vi "Intan_Update_XY_AxisLims.vi"(0 "NscansRead":i32, 1 "offset factor":dbl=1.0, 5 "FS (Hz)":dbl, 7 "XscaleClusterCurrent":T1, 9 "DisplayLength(s)":dbl, 11 "DT_scale (s)":dbl, 12 "Nchans to Display":i16) -> (4 "XscaleRollover":bool, 6 "DispLengthChanged":bool, 8 "offsetChanged":bool, 10 "NchansChanged":bool, 14 "XYlims Update Cluster":T2, 15 "UpdateCode":i16)   [LabVIEW 2017]
panel:
  out "Nupdates":dbl
  out "samps displayed":i64
  out "newXoffset":dbl
  out "YscaleMinOut":dbl
  out "YscaleMax_Out":dbl
  out "XscaleOffsetOut":dbl
  out "XscaleMaxOut":dbl
  out "XscaleMinOut":dbl
  out "Time since last update (s)":dbl
  out "NsampsSinceScrnUpdate":i64
  out "Nsamps refresh":dbl
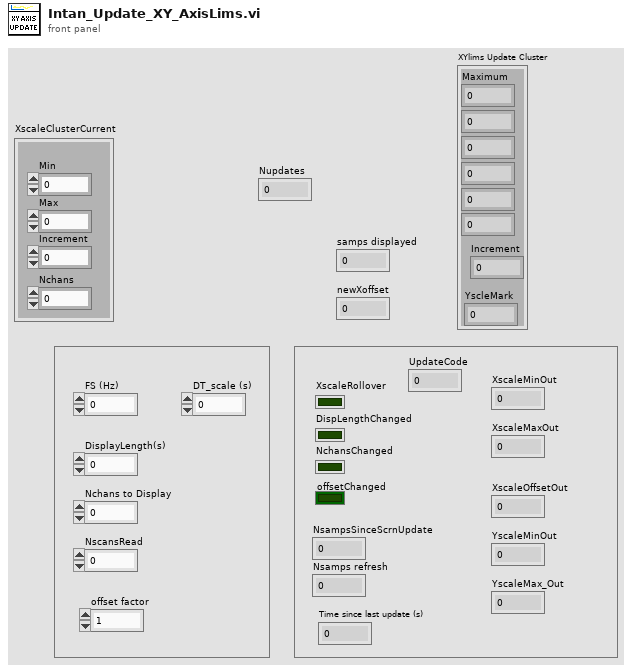
[diagram p1: front panel]
types:
  T1 = cluster{"Min":dbl, "Max":dbl, "Increment":dbl, "Nchans":dbl}
  T2 = cluster{"Maximum":dbl, dbl, dbl, dbl, dbl, dbl, "YscleMark":dbl, "Increment":dbl}
  T3 = cluster{"Max":dbl, dbl, dbl, dbl, dbl, dbl, dbl, "Increment":dbl}
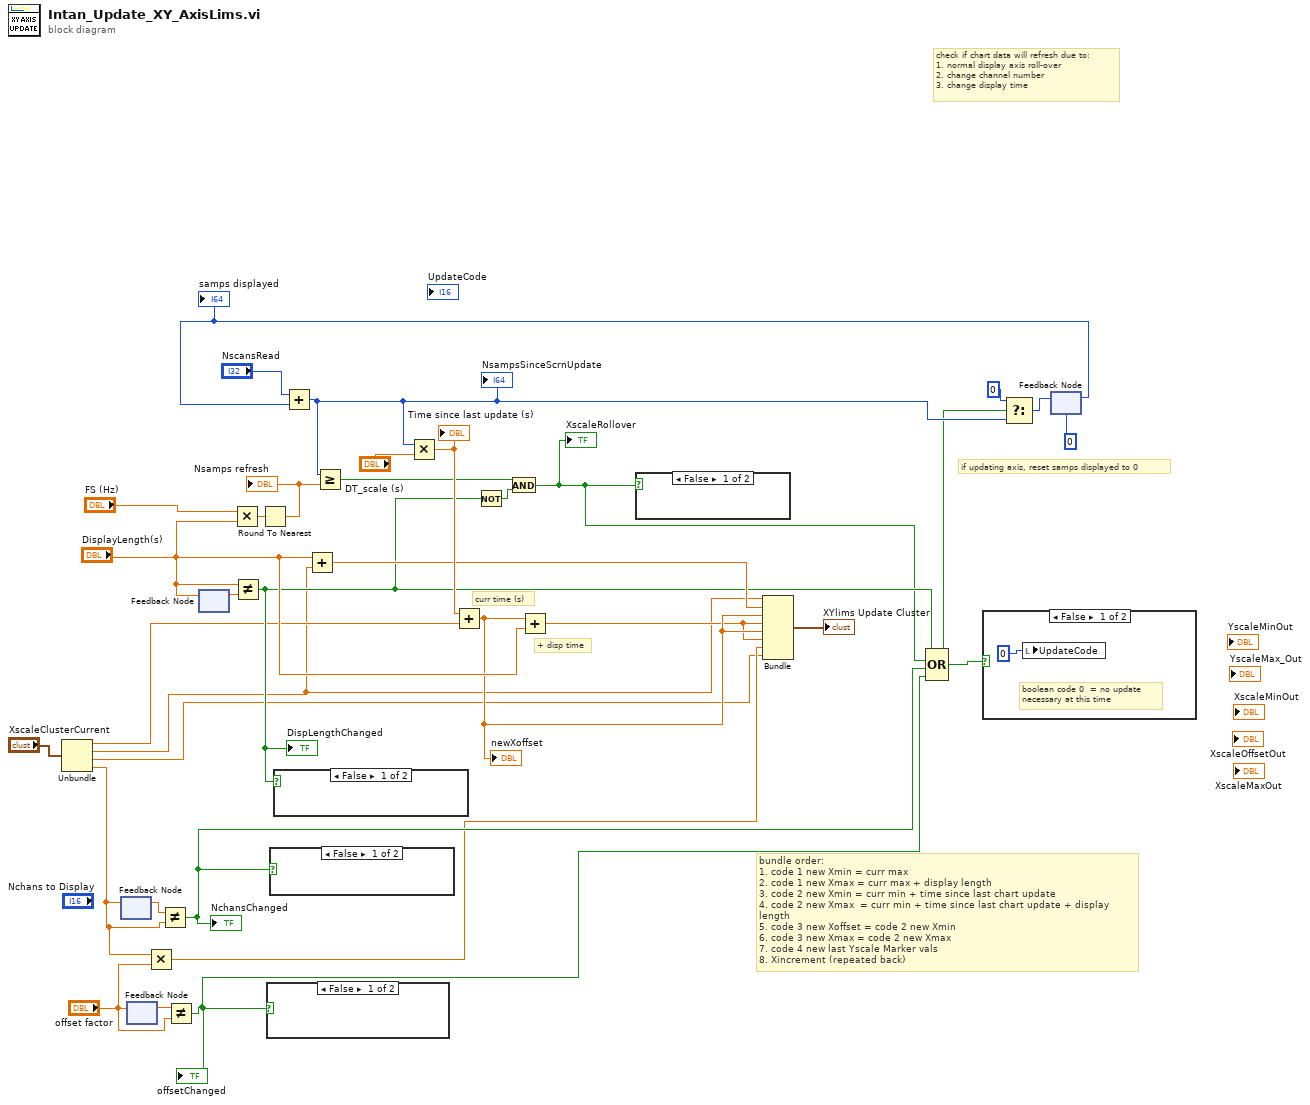
[diagram p0: block diagram]
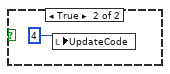
[diagram p2: hidden frame]
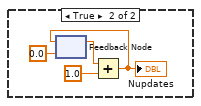
[diagram p3: hidden frame]
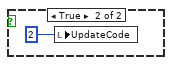
[diagram p4: hidden frame]
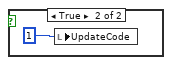
[diagram p5: hidden frame]
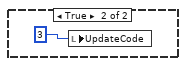
[diagram p6: hidden frame]
diagram:
  # "if updating axis, reset samps displayed to 0"
  # "bundle order: \n1. code 1 new Xmin = curr max\n2. code 1 new Xmax = curr max + display length\n3. code 2 new Xmin = curr min + time since last chart update\n4. code 2 new Xmax  = curr min + time since last chart update + display length\n5. code 3 new Xoffset = code 2 new Xmin\n6. code 3 new Xmax = code 2 new Xmax\n7. code 4 new last Yscale Marker vals\n8. Xincrement (repeated back)"
  # "+ disp time"
  # "curr time (s)"
  # "check if chart data will refresh due to:\n1. normal display axis roll-over\n2. change channel number\n3. change display time"
  n1 = Unbundle("XscaleClusterCurrent") -> ("Min"=w4:dbl, "Max"=w3:dbl, "Increment"=w2:dbl, "Nchans"=w1:dbl)
  n2 = feedback #1() -> (w22:dbl)  [unwired: 1 in]
  n3 = feedback-in #1(w1) -> ()
  n4 = feedback #2() -> (w11:dbl)  [unwired: 1 in]
  n5 = feedback-in #2("offset factor") -> ()
  n6 = Multiply(x=w1, y="offset factor") -> (x*y=w7:dbl)
  n7 = Not Equal?(x=w22, y=w1) -> (x != y?=w10:bool)
  "NchansChanged" <- w10
  n8 = Not Equal?(x=w11, y="offset factor") -> (x != y?=w9:bool)
  "offsetChanged" <- w9
  n9 = feedback #3() -> (w30:dbl)  [unwired: 1 in]
  n10 = feedback-in #3("DisplayLength(s)") -> ()
  n11 = Multiply(x="FS (Hz)", y="DisplayLength(s)") -> (x*y=w33:dbl)
  n12 = Not Equal?(x="DisplayLength(s)", y=w30) -> (x != y?=w13:bool)
  "DispLengthChanged" <- w13
  n13 = Round To Nearest(number=w33) -> (nearest integer value=w32:dbl)
  "Nsamps refresh" <- w32
  n14 = case shown="False" w9 {
    frame False {
    }
    frame True {
      n15 = local write "UpdateCode"(i16 4 ("UpdateCode")) -> ()
    }
  }
  n16 = case shown="False" w10 {
    frame False {
    }
    frame True {
      n17 = local write "UpdateCode"(i64 3 ("y")) -> ()
    }
  }
  n18 = case shown="False" w13 {
    frame False {
    }
    frame True {
      n19 = local write "UpdateCode"(i64 2 ("y")) -> ()
    }
  }
  n20 = Add(x="DisplayLength(s)", y=w3) -> (x+y=w16:dbl)
  n21 = Not(x=w13) -> (.not. x?=w29:bool)
  n22 = feedback #4(i64 0 ("y")) -> (w19:i64)
  "samps displayed" <- w19
  n23 = Add(x="NscansRead", y=w19) -> (x+y=w28:i64)
  "NsampsSinceScrnUpdate" <- w28
  n24 = Greater Or Equal?(x=w28, y=w32) -> (x >= y?=w21:bool)
  n25 = Multiply(x=w28, y="DT_scale (s)") -> (x*y=w27:dbl)
  "Time since last update (s)" <- w27
  n26 = Add(x=w27, y=w4) -> (x+y=w15:dbl)
  "newXoffset" <- w15
  n27 = And(x=w21, y=w29) -> (x .and. y?=w12:bool)
  "XscaleRollover" <- w12
  n28 = Add(x=w15, y="DisplayLength(s)") -> (x+y=w14:dbl)
  n29 = case shown="False" w12 {
    frame False {
    }
    frame True {
      n30 = local write "UpdateCode"(u16 1 ("y")) -> ()
    }
  }
  n31 = Bundle("Max"=w3, w16, w15, w14, w15, w14, w7, "Increment"=w2) -> (→"XYlims Update Cluster":T3)  [unwired: 1 in]
  n32 = Compound Arithmetic op=OR(w12, w13, w10, w9) -> (w17:bool)
  n33 = case shown="False" w17 {
    frame False {
      # "boolean code 0  = no update\nnecessary at this time"
      n34 = local write "UpdateCode"(u16 0 ("y")) -> ()
    }
    frame True {
      n35 = feedback #5(0.0 ("Nupdates")) -> (w41:dbl)
      n36 = Add(x=w41, y=1.0) -> (x+y=w39:dbl)
      "Nupdates" <- w39
      n37 = feedback-in #5(w39) -> ()
    }
  }
  n38 = Select(t=i64 0 ("y"), s=w17, f=w28) -> (s? t:f=w20:i64)
  n39 = feedback-in #4(w20) -> ()
